vi "Test Copy Image to Pixmap With Mask ARGB.vi"(8 "error in (no error)":errorcluster, 11 "Test Case In":refnum<class "Image.lvclass">) -> (0 "error out":errorcluster, 3 "Test Case Out":refnum<class "Image.lvclass">)   [LabVIEW 2020, in "g_ar_toolkit.test.lvlib" / "Image.lvclass"]
uses:
  Image.lvclass
  C:/Program Files (x86)/National Instruments/LabVIEW 2020/vi.lib/Astemes/LUnit/Test Case.lvclass
  g_ar_toolkit.common/Image Size (Integer).ctl
  <vilib>/Astemes/LUnit/Test Case.lvclass/Test Case.ctl
  g_ar_toolkit.image/MaskFromColour.vi
  g_ar_toolkit.image/CopyImageToPixmapARGBWithMask.vi
  4993e8ee-a06a-463a-9684-69129f64d5ce.vi
  g_ar_toolkit.image/CreateEmptyImageGreyscale.vi/6598b9e0-8a08-46f5-91fd-ca1b87217137.vi
  g_ar_toolkit.image/Create Image.vi
  g_ar_toolkit.image/CreateEmptyImageARGB.vi
  g_ar_toolkit.image/Copy Array to Image.vi
  g_ar_toolkit.image/CopyArrayToImageARGB.vi
  g_ar_toolkit.image/MaskFromColour.vi/5701baee-35e2-4306-9a77-a9fdbb5b3a7f.vi
  g_ar_toolkit.image/BitwiseNOTGreyscale.vi/f9ee80d6-438b-4cfb-91f1-04b98ac80474.vi
  g_ar_toolkit.image/CopyImageToPixmapARGBWithMask.vi/5c639587-cf36-4d54-93d9-e654c7c24c6e.vi
  <vilib>/Astemes/LUnit/Append Pass Result.vi
  <vilib>/Astemes/LUnit/Append Fail Result.vi
  <vilib>/Astemes/LUnit/Describe Comparison.vi
  <vilib>/Astemes/LUnit/Compare Variants.vi
  g_ar_toolkit.image/CreateEmptyImageARGB.vi/3321fa97-f432-4e1e-8db9-a0df79aed21b.vi
  g_ar_toolkit.image/ARGBColourToU32.vi
  g_ar_toolkit.image/CopyArrayToImageARGB.vi/2ca5c3f0-e0c8-4997-b936-d846b6ef5cb6.vi
  <vilib>/Astemes/LUnit/Run In UI.vi
  <vilib>/Utility/error.llb/Clear Errors.vi
  g_ar_toolkit.common/Module Path.vi
  <vilib>/Utility/error.llb/Error Cluster From Error Code.vi
  <vilib>/picture/pixmap.llb/Flatten Pixmap.vi
  <vilib>/Astemes/LUnit/Describe Variant.vi
  g_ar_toolkit.common/g_ar_toolkit.common.lvlib
  g_ar_toolkit.image/g_ar_toolkit.image.lvlib
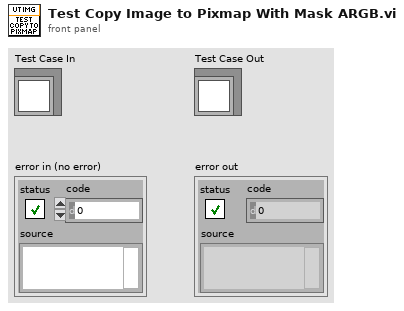
[diagram p1: front panel]
types:
  T1 = typedef "g_ar_toolkit.common.lvlib/Image Size (Integer).ctl" = cluster{"Width":u16, "Height":u16}
  T2 = typedef "imagedata.ctl" = cluster{"image type":i32, "image depth":i32, "image":u8[], "mask":u8[], "colors":u32[], "Rectangle":cluster{"left":i16, "top":i16, "right":i16, "bottom":i16}}
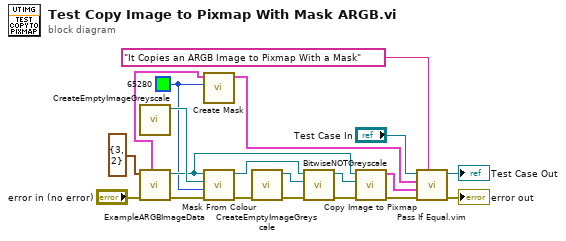
[diagram p0: block diagram]
diagram:
  w1 = u32 65280 ("RGB")
  n1 = call "CreateEmptyImageGreyscale.vi"() -> ("New Greyscale Image"=w14:refnum<data-value>)  [unwired: 10 in, 1 out]
  n2 = call "ExampleARGBImageData.vi"("error in (no error)"="error in (no error)", "Image Size"=T1 {"Width"=3, "Height"=2} ("Preallocated Image Size (Default - 0,0)")) -> ("error out"=w12:errorcluster, "Data Value Reference out"=w13:refnum<data-value>, "ARGB Pixmap Data"=w15:T2)  [unwired: 6 in, 1 out]
  n3 = call <vilib>:"Create Mask.vi"("Mask Color (Black)"=w1, "image data"=w15) -> ("image data"=w5:T2)  [unwired: 9 in]
  n4 = call-poly "Mask From Colour.vi"("error in (no error)"=w12, "Value"=w1, "Mask Destination"=w14, "ARGB Image Source"=w13) -> ("error out"=w4:errorcluster, "Mask Destination (duplicate)"=w8:refnum<data-value>)  [unwired: 6 in]
  n5 = call "CreateEmptyImageGreyscale.vi"("error in (no error)"=w4) -> ("error out"=w3:errorcluster, "New Greyscale Image"=w7:refnum<data-value>)  [unwired: 9 in]
  n6 = call "BitwiseNOTGreyscale.vi"("error in (no error)"=w3, "Greyscale Image Destination"=w7, "Greyscale Image Source"=w8) -> ("error out"=w9:errorcluster, "Greyscale Image Destination (duplicate)"=w2:refnum<data-value>)  [unwired: 7 in]
  n7 = call-poly "Copy Image to Pixmap.vi"("error in (no error)"=w9, "Greyscale Mask"=w2, "ARGB Image Source"=w13) -> ("error out"=w10:errorcluster, "Pixmap Image Data"=w6:T2)  [unwired: 7 in]
  n8 = call "Pass If Equal.vim"("Description"="It Copies an ARGB Image to Pixmap With a Mask", "error in (no error)"=w10, "Actual"=w6, "Expected"=w5, "LUnit Test Case In"="Test Case In") -> ("error out"=→"error out":errorcluster, "LUnit Test Case Out"=→"Test Case Out":refnum<class "Image.lvclass">)  [unwired: 5 in]
